vi "Ch1-Ex3.vi"() -> ()   [LabVIEW 2018]
panel:
  out "Array":dbl[](array[numeric])
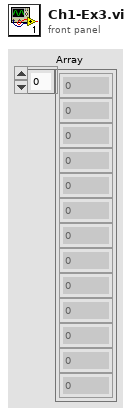
[diagram p1: front panel]
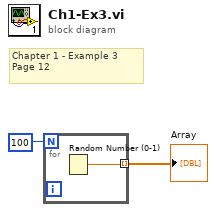
[diagram p0: block diagram]
diagram:
  # "Chapter 1 - Example 3\nPage 12"
  n1 = for {
    N: 100 -> [_]
    tunnel: [w3] -> w1 mode=indexing
    n2 = Random Number (0-1)() -> (number: 0 to 1=w3:dbl)
  }
  "Array" <- w1
